vi "CAN Send.vi"(8 "error in (no error)":errorcluster, 9 "data":u8[](array[numeric]), 10 "messageID":u32 format="%.0x") -> (0 "error out":errorcluster)   [LabVIEW 2009, in "CAN.lvlib"]
uses:
  CAN.lvlib
  Serial.lvlib
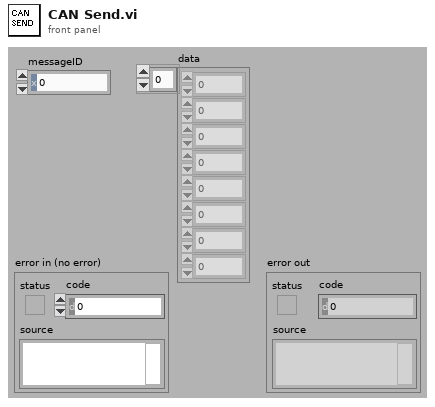
[diagram p1: front panel]
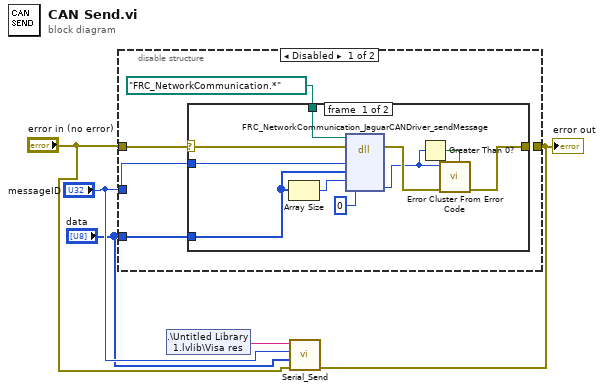
[diagram p0: block diagram]
diagram:
  n1 = shared-variable ".\\Untitled Library 1.lvlib\\Visa res"() -> (w5:string)  [unwired: 1 in, 1 out]
  n2 = call "Serial_Send.vi"("error in"="error in (no error)", "data"="data", "messageID"="messageID", "VISA resource name"=w5) -> ("error out"=w1:errorcluster)  [unwired: 6 in, 1 out]
  "error out" <- w1
  n3 = disable-structure shown="Disabled" {
    disable-tunnel: "error in (no error)" -> [w8 _]
    disable-tunnel: w1 -> [_ _]
    disable-tunnel: "messageID" -> [w7 _]
    disable-tunnel: "data" -> [w6 _]
    frame #0 {
      n4 = case shown="No Error" w8 {
        selector: w8 -> [w16 w20]
        tunnel: path "FRC_NetworkCommunication.*" ("path in") -> [w19 _]
        tunnel: [w12 w20] -> _
        tunnel: w7 -> [w11 _]
        tunnel: w6 -> [w10 _]
        frame #0 {
          n5 = Array Size(array=w10) -> (size(s)=w17:i32)
          n6 = dll-call lib="?" fn="FRC_NetworkCommunication_JaguarCANDriver_sendMessage"(path in=w19, error in=w16, "messageID"=w11, "data"=w10, "dataSize"=w17, "status"=0) -> (error out=w15:errorcluster, "status"=w13:i32)  [unwired: 3 in, 3 out]
          n7 = Greater Than 0?(x=w13) -> (x > 0?=w14:bool)
          n8 = call <vilib>:"Error Cluster From Error Code.vi"("is warning? (False)"=w14, "error in (no error)"=w15, "error code (0)"=w13) -> ("error out"=w12:errorcluster)  [unwired: 1 in, 5 out]
        }
        frame #1 {
        }
      }
    }
    frame #1 {
    }
  }
